vi "BeltStall.vi"(1 "Boolean":bool, 2 "BeltSpeed":dbl) -> (0 "BeltSpeedOut":dbl)   [LabVIEW 2016]
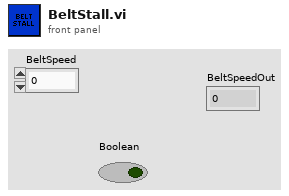
[diagram p1: front panel]
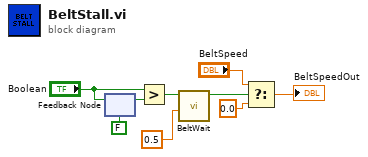
[diagram p0: block diagram]
diagram:
  n1 = feedback-in #1("Boolean") -> ()
  n2 = feedback #1(FALSE ("Boolean")) -> (w9:bool)
  n3 = Greater?(x="Boolean", y=w9) -> (0:w6:bool)
  n4 = call "BeltWait.vi"("Target Time (s)"=0.5 ("y"), "First Time?"=w6) -> ("Completed"=w1:bool)  [unwired: 8 in, 1 out]
  n5 = Select(t="BeltSpeed", s=w1, f=0.0) -> (s? t:f=→"BeltSpeedOut":dbl)
